vi "b-fields many sensors from orbit.vi"(10 "orbit magnetic field data":T1 {"omega" format="%#_13g"}, 11 "orbit parameters":T3) -> (1 "derivatives":dbl[][](array[numeric]), 2 "measured field":dbl[](array[numeric]), 3 "predicted field":dbl[](array[numeric]), 4 "predicted location":dbl[][](array[numeric]), 5 "sensor0 measured":dbl[][](array[numeric]), 7 "sensor0 prediction":dbl[][](array[numeric]))   [LabVIEW 2017]
uses:
  typedefs/orbit parameters full.ctl
  typedefs/orbit magnetic field data.ctl
  typedefs/magnetomter reading set.ctl
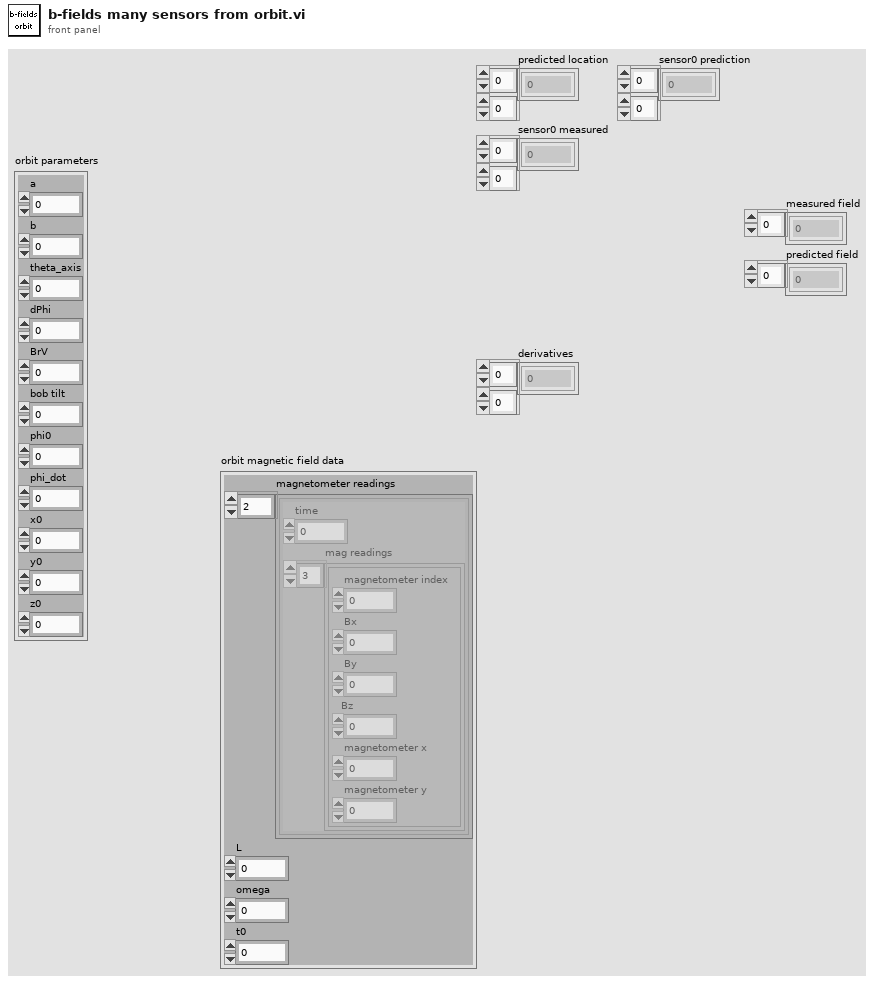
[diagram p1: front panel]
types:
  T1 = typedef "orbit magnetic field data.ctl" = cluster{"magnetometer readings":T2[], "L":dbl, "omega":dbl, "t0":fxp<+,48,48>}
  T2 = typedef "magnetomter reading set.ctl" = cluster{"time":fxp<+,48,48>, "mag readings":cluster{"magnetometer index":dbl, "Bx":dbl, "By":dbl, "Bz":dbl, "magnetometer x":dbl, "magnetometer y":dbl}[]}
  T3 = typedef "orbit parameters full.ctl" = cluster{"a":dbl, "b":dbl, "theta_axis":dbl, "dPhi":dbl, "BrV":dbl, "bob tilt":dbl, "phi0":dbl, "phi_dot":dbl, "x0":dbl, "y0":dbl, "z0":dbl}
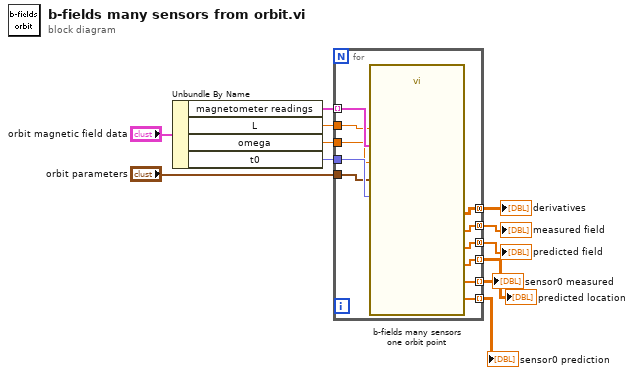
[diagram p0: block diagram]
diagram:
  n1 = Unbundle By Name("orbit magnetic field data") -> ("magnetometer readings"=w7:T2[], "L"=w6:dbl, "omega"=w5:dbl, "t0"=w4:fxp<+,48,48>)
  n2 = for {
    tunnel: w7 -> [w23] mode=indexing
    tunnel: w4 -> [w22]
    tunnel: "orbit parameters" -> [w21]
    tunnel: [w20] -> w10 mode=concatenating
    tunnel: [w19] -> w9 mode=concatenating
    tunnel: [w18] -> w11 mode=concatenating
    tunnel: w6 -> [w17]
    tunnel: w5 -> [w16]
    tunnel: [w15] -> w3 mode=indexing
    tunnel: [w14] -> w2 mode=indexing
    tunnel: [w13] -> w1 mode=indexing
    n3 = call "b-fields many sensors one orbit point.vi"("t0"=w22, "omega"=w16, "L"=w17, "magnetometer readings"=w23, "orbit parameters"=w21) -> ("measured field"=w20:dbl[], "derivatives"=w18:dbl[][], "predicted field"=w19:dbl[], "predicted location"=w15:dbl[], "sensor0 prediction"=w13:dbl[], "sensor0 measured"=w14:dbl[])  [unwired: 1 in]
  }
  "measured field" <- w10
  "predicted field" <- w9
  "derivatives" <- w11
  "predicted location" <- w3
  "sensor0 measured" <- w2
  "sensor0 prediction" <- w1
